vi "DHE_GetImageParams.vi"() -> (1 "image string":string, 2 "DHE_IMAGE":T1={"title"="", "comment"="", "rootname"="/uyq0/home/bonati/junk", "imnumber"=2, "mext"=FALSE, "imdir"="uyq0/home/bonati", "basename"="junk", "imprefix"="_none_", "imsufix"="_none_", "froot"="/"})   [LabVIEW 2016]
uses:
  private/vis/DHE_Img.ctl
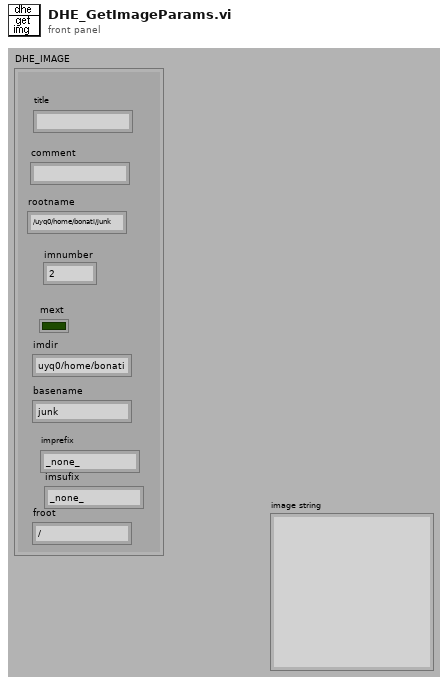
[diagram p1: front panel]
types:
  T1 = typedef "DHE_Img.ctl" = cluster{"title":string, "comment":string, "rootname":string, "imnumber":i32, "mext":bool, "imdir":string, "basename":string, "imprefix":string, "imsufix":string, "froot":string}
  T2 = typedef "DatabaseHand_RefNum.ctl" = refnum<vi>
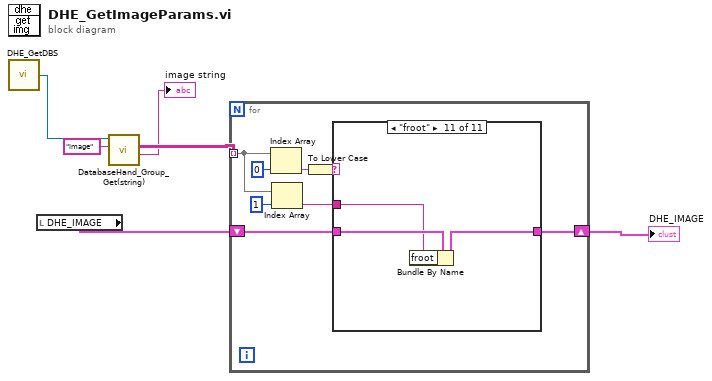
[diagram p0: block diagram]
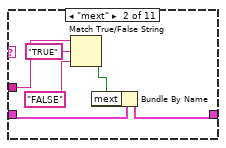
[diagram p3: hidden frame]
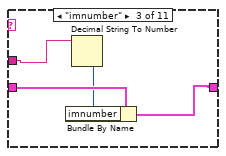
[diagram p4: hidden frame]
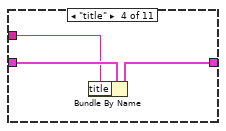
[diagram p5: hidden frame]
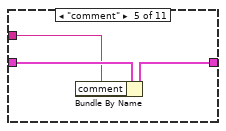
[diagram p6: hidden frame]
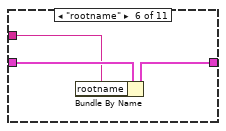
[diagram p7: hidden frame]
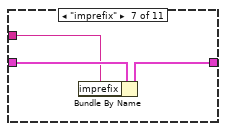
[diagram p8: hidden frame]
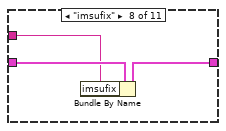
[diagram p9: hidden frame]
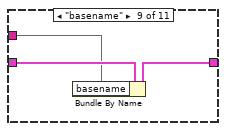
[diagram p10: hidden frame]
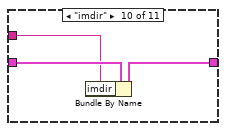
[diagram p11: hidden frame]
diagram:
  n1 = call "DHE_GetDBS.vi"() -> ("DHE_DBSRef"=w1:T2)  [unwired: 9 out]
  n2 = local read "DHE_IMAGE"() -> (w3:T1)
  n3 = call "DatabaseHand_Group_Get(string).vi"("group"="image", "Database RefNum in"=w1) -> ("group string"=→"image string":string, "group array"=w5:string[][])  [unwired: 1 in, 7 out]
  n4 = for {
    tunnel: w5 -> [w9] mode=indexing
    shift-right: [w11] -> w4
    shift-left: w3 -> [w12]
    n5 = Index Array(array=w9, index=0) -> (element=w13:string)
    n6 = Index Array(array=w9, index=1) -> (element=w8:string)
    n7 = To Lower Case(string=w13) -> (all lower case string=w7:string)
    n8 = case shown="\"froot\"" w7 {
      tunnel: w12 -> [w15 w21 w25 w28 w31 w34 w37 w40 w43 w46 w49]
      tunnel: [w15 w20 w24 w27 w30 w33 w36 w39 w42 w45 w48] -> w11
      tunnel: w8 -> [_ w19 w23 w26 w29 w32 w35 w38 w41 w44 w47]
      frame Default {
      }
      frame "mext" {
        n9 = Match True/False String(2:"FALSE" ("false string"), 3:"TRUE" ("true string"), 4:w19) -> (0:w18:bool)  [unwired: 1 out]
        n10 = Bundle By Name(cluster=w21, "mext"=w18) -> (w20:T1)
      }
      frame "imnumber" {
        n11 = Decimal String To Number(string=w23) -> (number=w22:i32)  [unwired: 3 out]
        n12 = Bundle By Name(cluster=w25, "imnumber"=w22) -> (w24:T1)
      }
      frame "title" {
        n13 = Bundle By Name(cluster=w28, "title"=w26) -> (w27:T1)
      }
      frame "comment" {
        n14 = Bundle By Name(cluster=w31, "comment"=w29) -> (w30:T1)
      }
      frame "rootname" {
        n15 = Bundle By Name(cluster=w34, "rootname"=w32) -> (w33:T1)
      }
      frame "imprefix" {
        n16 = Bundle By Name(cluster=w37, "imprefix"=w35) -> (w36:T1)
      }
      frame "imsufix" {
        n17 = Bundle By Name(cluster=w40, "imsufix"=w38) -> (w39:T1)
      }
      frame "basename" {
        n18 = Bundle By Name(cluster=w43, "basename"=w41) -> (w42:T1)
      }
      frame "imdir" {
        n19 = Bundle By Name(cluster=w46, "imdir"=w44) -> (w45:T1)
      }
      frame "froot" {
        n20 = Bundle By Name(cluster=w49, "froot"=w47) -> (w48:T1)
      }
    }
  }
  "DHE_IMAGE" <- w4
